vi "Calc Frequency-RMS-Pk-Pk.vi"(0 "Signal Data In":sgl[](array[numeric]), 1 "Sample Rate":dbl) -> (15 "RMS":dbl[](array[numeric]), 16 "Pk-Pk":dbl[](array[numeric]), 17 "Frequency":dbl[](array[numeric]), 18 "Peak":dbl[](array[numeric]), 19 "Valley":dbl[](array[numeric]))   [LabVIEW 2019]
uses:
  <vilib>/Analysis/3filter.llb/Savitzky-Golay Filter (DBL).vi
  <vilib>/Analysis/baseanly.llb/Mean (DBL).vi
  <vilib>/ptbypt/NI_PtbyPt.lvlib
  <vilib>/Analysis/NI_AALBase.lvlib
panel:
  out "Waveform Chart 2":dbl[](graph)
  out "Waveform Chart":dbl[][](graph)
  # "362mv +/- 90mv"
  # "0"
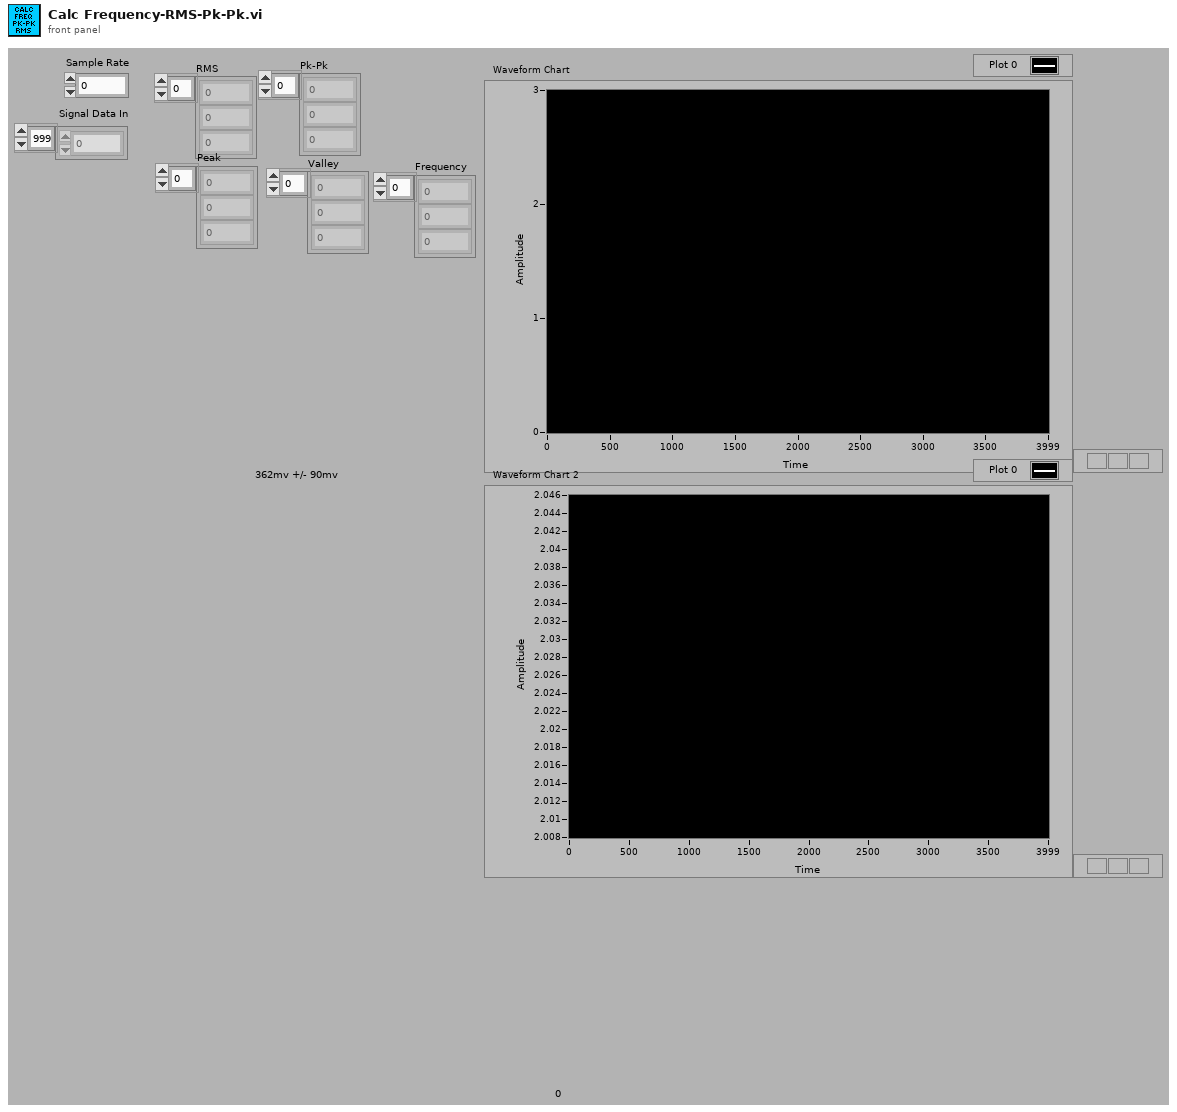
[diagram p1: front panel]
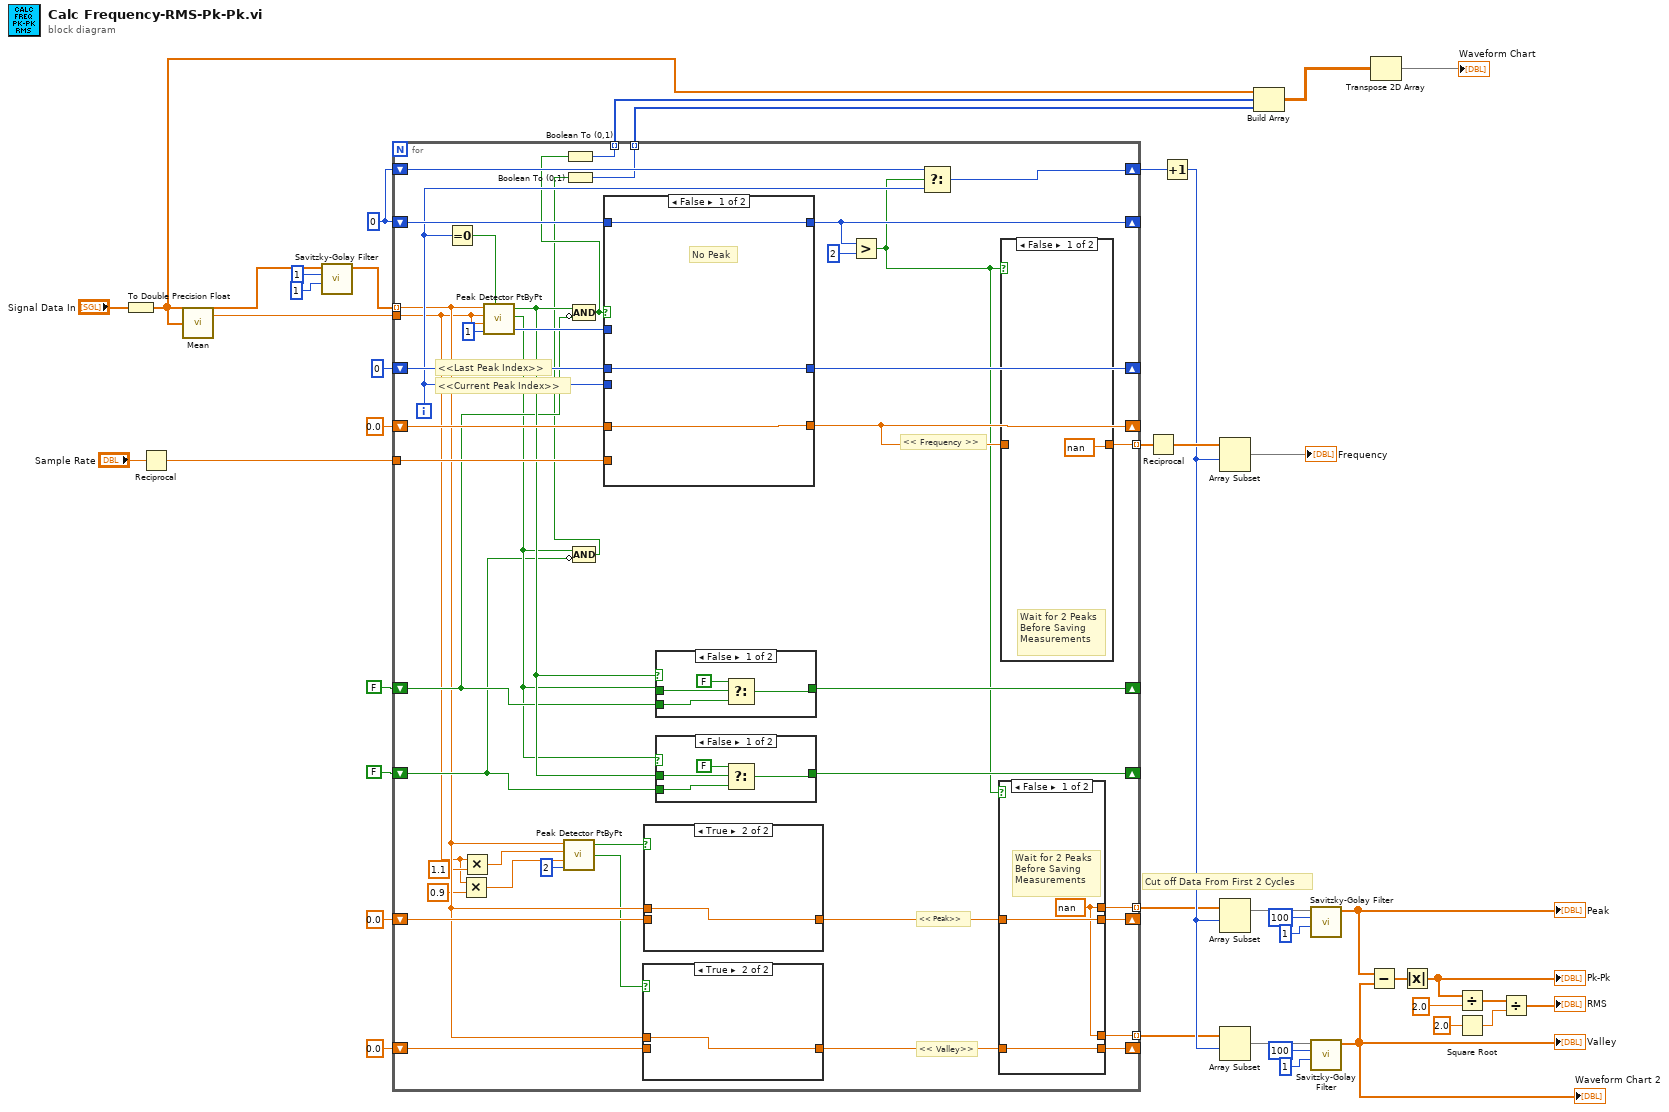
[diagram p0: block diagram]
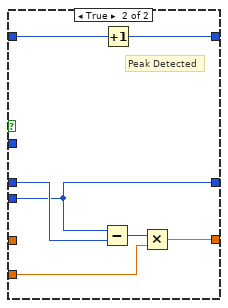
[diagram p8: hidden frame]
diagram:
  w35 = 0
  # "Cut off Data From First 2 Cycles"
  n1 = To Double Precision Float(number="Signal Data In") -> (double precision float=w5:dbl[])
  n2 = Reciprocal(x="Sample Rate") -> (1/x=w37:dbl)
  n3 = call-poly <vilib>:"Mean.vi"("X"=w5) -> ("mean"=w33:dbl)  [unwired: 1 out]
  n4 = call-poly <vilib>:"Savitzky-Golay Filter.vi"("polynomial order"=1, "side points"=1, "X"=w5) -> ("Filtered X"=w4:dbl[])  [unwired: 7 in, 1 out]
  n5 = for {
    tunnel: w4 -> [w49] mode=indexing
    shift-right: [w75] -> _
    shift-left: 0 -> [w83]
    tunnel: w37 -> [w82]
    shift-right: [w80] -> _
    shift-left: 0.0 -> [w81]
    tunnel: [w79] -> w38 mode=indexing
    shift-right: [w77] -> _
    shift-left: w35 -> [w78]
    shift-right: [w72] -> w34
    shift-left: w35 -> [w73]
    tunnel: w33 -> [w44]
    tunnel: [w71] -> w30 mode=indexing
    tunnel: [w70] -> w28 mode=indexing
    shift-right: [w68] -> _
    shift-left: FALSE -> [w64]
    shift-right: [w67] -> _
    shift-left: FALSE -> [w62]
    shift-right: [w56] -> _
    shift-left: 0.0 -> [w58]
    tunnel: [w55] -> w22 mode=indexing
    shift-right: [w53] -> _
    shift-left: 0.0 -> [w54]
    tunnel: [w52] -> w20 mode=indexing
    i -> [w74]
    # "<< Valley>>"
    # "<< Peak>>"
    # "<<Last Peak Index>>"
    # "<<Current Peak Index>>"
    # "<< Frequency >>"
    n6 = Equal To 0?(x=w74) -> (x = 0?=w84:bool)
    n7 = Multiply(x=w44, y=0.9) -> (x*y=w43:dbl)
    n8 = Multiply(x=w44, y=1.1) -> (x*y=w42:dbl)
    n9 = call <vilib>:"Peak Detector PtByPt.vi"("x"=w49, "threshold peak"=w44, "threshold valley"=w44, "width"=1, "initialize"=w84) -> ("peak"=w66:bool, "valley"=w63:bool, "error"=w69:i32)
    n10 = call <vilib>:"Peak Detector PtByPt.vi"("x"=w49, "threshold peak"=w42, "threshold valley"=w43, "width"=2) -> ("peak"=w59:bool, "valley"=w48:bool)  [unwired: 1 in, 1 out]
    n11 = Compound Arithmetic op=AND(w66, invert w64) -> (w65:bool)
    n12 = Boolean To (0,1)(Boolean=w65) -> (0, 1=w71:i16)
    n13 = Compound Arithmetic op=AND(w63, invert w62) -> (w61:bool)
    n14 = Boolean To (0,1)(Boolean=w61) -> (0, 1=w70:i16)
    n15 = case shown="False" w65 {
      tunnel: [w108 w109] -> w75
      tunnel: w74 -> [_ w109]
      tunnel: w83 -> [w108 w112]
      tunnel: w82 -> [_ w114]
      tunnel: [w107 w113] -> w80
      tunnel: w81 -> [w107 _]
      tunnel: [w106 w110] -> w77
      tunnel: w78 -> [w106 w111]
      tunnel: w69 -> [_ _]
      frame False {
        # "No Peak"
      }
      frame True {
        # "Peak Detected"
        n16 = Subtract(x=w109, y=w112) -> (x-y=w115:i32)
        n17 = Increment(x=w111) -> (x+1=w110:i32)
        n18 = Multiply(x=w115, y=w114) -> (x*y=w113:dbl)
      }
    }
    n19 = case shown="True" w48 {
      tunnel: w49 -> [_ w86]
      tunnel: [w85 w86] -> w47
      tunnel: w54 -> [w85 _]
      frame False {
      }
      frame True {
      }
    }
    n20 = case shown="True" w59 {
      tunnel: w49 -> [_ w93]
      tunnel: [w92 w93] -> w51
      tunnel: w58 -> [w92 _]
      frame False {
      }
      frame True {
      }
    }
    n21 = case shown="False" w66 {
      selector: w66 -> [_ w103]
      tunnel: [w99 w103] -> w68
      tunnel: w63 -> [w102 _]
      tunnel: w64 -> [w100 _]
      frame False {
        n22 = Select(t=FALSE, s=w102, f=w100) -> (s? t:f=w99:bool)
      }
      frame True {
      }
    }
    n23 = case shown="False" w63 {
      selector: w63 -> [_ w98]
      tunnel: [w94 w98] -> w67
      tunnel: w66 -> [w97 _]
      tunnel: w62 -> [w95 _]
      frame False {
        n24 = Select(t=FALSE, s=w97, f=w95) -> (s? t:f=w94:bool)
      }
      frame True {
      }
    }
    n25 = Greater?(x=w77, y=2) -> (0:w57:bool)
    n26 = Select(t=w73, s=w57, f=w74) -> (s? t:f=w72:i32)
    n27 = case shown="False" w57 {
      tunnel: w51 -> [w89 w91]
      tunnel: [w89 w91] -> w56
      tunnel: [w87 w91] -> w55
      tunnel: w47 -> [w88 w90]
      tunnel: [w88 w90] -> w53
      tunnel: [w87 w90] -> w52
      frame False {
        w87 = nan
        # "Wait for 2 Peaks\nBefore Saving\nMeasurements"
      }
      frame True {
        # "More then 2\nCycles Detected"
      }
    }
    n28 = case shown="False" w57 {
      tunnel: w80 -> [_ w105]
      tunnel: [nan w105] -> w79
      frame False {
        # "Wait for 2 Peaks\nBefore Saving\nMeasurements"
        # "Wait for 2 Peaks\nBefore Saving\nMeasurements"
      }
      frame True {
        # "More then 2\nCycles Detected"
      }
    }
  }
  n29 = Reciprocal(x=w38) -> (1/x=w32:dbl[])
  n30 = Increment(x=w34) -> (x+1=w31:i32)
  n31 = Array Subset(array=w32, index=w31) -> (→"Frequency":dbl[])  [unwired: 1 in]
  n32 = Array Subset(array=w22, index=w31) -> (w9:dbl[])  [unwired: 1 in]
  n33 = Array Subset(array=w20, index=w31) -> (w2:dbl[])  [unwired: 1 in]
  n34 = Build Array(w5, w30, w28) -> (w21:dbl[][])
  n35 = call-poly <vilib>:"Savitzky-Golay Filter.vi"("polynomial order"=1, "side points"=100, "X"=w9) -> ("Filtered X"=w3:dbl[])  [unwired: 7 in, 1 out]
  "Peak" <- w3
  n36 = call-poly <vilib>:"Savitzky-Golay Filter.vi"("polynomial order"=1, "side points"=100, "X"=w2) -> ("Filtered X"=w1:dbl[])  [unwired: 7 in, 1 out]
  "Valley" <- w1
  "Waveform Chart 2" <- w1
  n37 = Subtract(x=w3, y=w1) -> (x-y=w19:dbl[])
  n38 = Transpose 2D Array(2D array=w21) -> (transposed array=→"Waveform Chart":dbl[][])
  n39 = Absolute Value(x=w19) -> (abs(x)=w18:dbl[])
  "Pk-Pk" <- w18
  n40 = Divide(x=w18, y=2.0) -> (x/y=w16:dbl[])
  n41 = Square Root(x=2.0) -> (sqrt(x)=w15:dbl)
  n42 = Divide(x=w16, y=w15) -> (x/y=→"RMS":dbl[])
